vi "test attributes file.vi"() -> ()   [LabVIEW 2014]
uses:
  <vilib>/userdefined/High Color/IMAQdx.ctl
  <vilib>/vision/driver/IMAQdx.llb/IMAQdx Camera Control Mode.ctl
  <vilib>/vision/driver/NI_Vision_Acquisition_Software.lvlib
panel:
  in  "Path":path
  out "error out":errorcluster
  in  "Camera Name":T1
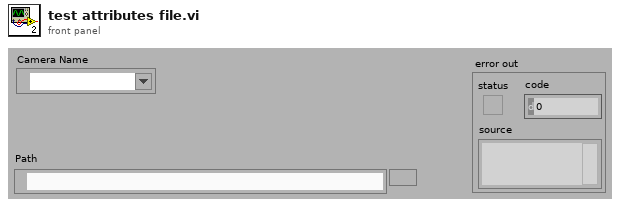
[diagram p1: front panel]
types:
  T1 = typedef "IMAQdx.ctl" = refnum<k21>
  T2 = typedef "NI_Vision_Acquisition_Software.lvlib/IMAQdx Camera Control Mode.ctl" = enum32{"Controller", "Listener"}
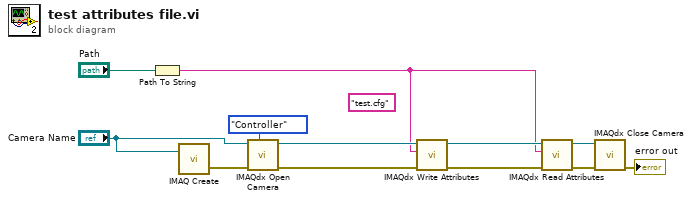
[diagram p0: block diagram]
diagram:
  (unwired) "test.cfg" ("Filename")
  n1 = Path To String(path="Path") -> (string=w1:string)
  n2 = call "IMAQ Create"("Image Name"="Camera Name") -> ("error out"=w12:errorcluster)  [unwired: 3 in, 2 out]
  n3 = call <vilib>:"IMAQdx Open Camera.vi"("Camera Control Mode"=IMAQdx_Camera_Control_Mode."Controller", "error in"=w12, "Session In"="Camera Name") -> ("error out"=w4:errorcluster, "Session Out"=w6:T1)  [unwired: 7 out]
  n4 = call <vilib>:"IMAQdx Write Attributes.vi"("error in"=w4, "Filename"=w1, "Session In"=w6) -> ("error out"=w3:errorcluster, "Session Out"=w5:T1)  [unwired: 7 in]
  n5 = call <vilib>:"IMAQdx Read Attributes.vi"("error in"=w3, "Filename"=w1, "Session In"=w5) -> ("error out"=w8:errorcluster, "Session Out"=w9:T1)  [unwired: 7 in]
  n6 = call <vilib>:"IMAQdx Close Camera.vi"("error in"=w8, "Session In"=w9) -> ("error out"=→"error out":errorcluster)  [unwired: 9 in]
